vi "Tcalc.vi"(1 "height":dbl=0.088, 2 "heave":dbl) -> (0 "appended array":T1)   [LabVIEW 2019]
uses:
  <vilib>/Analysis/Matrix/Datatypes/RealMatrix.ctl
  <vilib>/Analysis/Matrix/NI_Matrix.lvlib
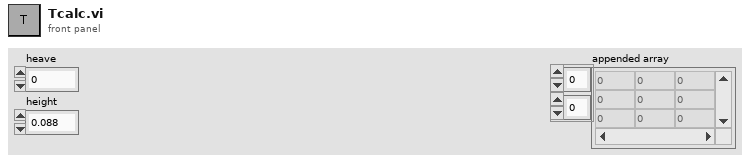
[diagram p1: front panel]
types:
  T1 = typedef "NI_Matrix.lvlib/RealMatrix.ctl" = dbl[][]
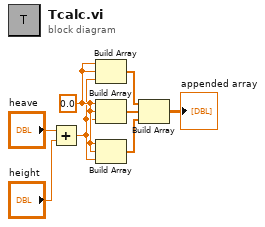
[diagram p0: block diagram]
diagram:
  w6 = 0.0 ("element")
  n1 = Add(x="heave", y="height") -> (x+y=w5:dbl)
  n2 = Build Array(w6, w6, w5) -> (w4:dbl[])
  n3 = Build Array(w6, w6, w5) -> (w3:dbl[])
  n4 = Build Array(w6, w6, w5) -> (w2:dbl[])
  n5 = Build Array(w4, w3, w2) -> (→"appended array":T1)
